vi "calc parameters.vi"(9 "Y start":dbl, 10 "basic params":T1={"X pixel #"=200, "X pixel size(um)"=1.0, "Y pixel #"=200, "Y pixel size(um)"=10.0, "line rate(Hz)"=1.0, "stage scan?"=FALSE} {"line rate(Hz)" min=1.0 max=2000.0 format="%#.3g"; "X pixel size(um)" min=0.0 max=10.0 format="%#.3g"; "X pixel #" min=2 max=20480 step=2 format="%#.3g"; "Y pixel size(um)" min=0.0 max=10.0 format="%#.3g"; "Y pixel #" min=2 max=204800 step=2 format="%#.3g"}) -> (1 "t":dbl, 2 "speed":dbl, 3 "Y end":dbl)   [LabVIEW 2015]
uses:
  type def/basic params.ctl
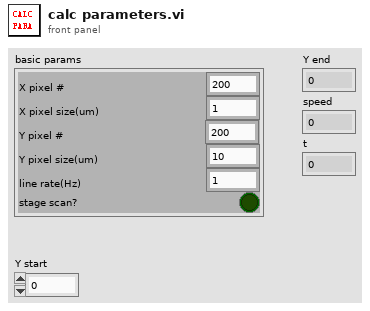
[diagram p1: front panel]
types:
  T1 = typedef "basic params.ctl" = cluster{"X pixel #":u32, "X pixel size(um)":dbl, "Y pixel #":u32, "Y pixel size(um)":dbl, "line rate(Hz)":dbl, "stage scan?":bool}
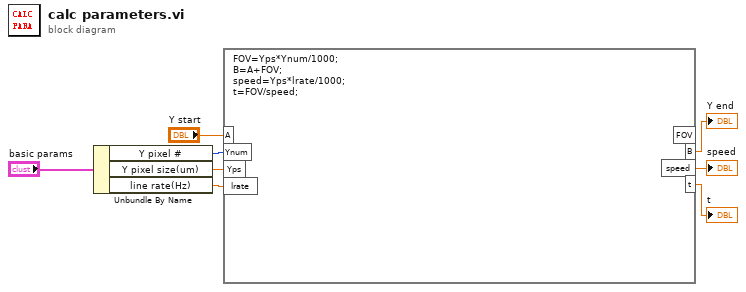
[diagram p0: block diagram]
diagram:
  n1 = Unbundle By Name("basic params") -> ("Y pixel #"=w5:u32, "Y pixel size(um)"=w4:dbl, "line rate(Hz)"=w3:dbl)
  n2 = formula code="FOV=Yps*Ynum/1000;\nB=A+FOV;\nspeed=Yps*lrate/1000;\nt=FOV/speed;"("A"="Y start", "Ynum"=w5, "Yps"=w4, "lrate"=w3) -> ("B"=→"Y end":dbl, "speed"=→"speed":dbl, "t"=→"t":dbl)  [unwired: 1 out]
